vi "_builtins_arrange_diagram.vi"(8 "error in (no error)":errorcluster, 10 "Arrange":T1, 11 "VI Refnum in":refnum<vi>) -> (0 "error out":errorcluster, 3 "VI Refnum out":refnum<vi>)   [LabVIEW 2019, in "Script.lvlib"]
doc: "Arranges the selected diagram objects according to horizontal position and adjacent terminal location.\n\nCreated by: Ryan Pacini"
uses:
  Script.lvlib
  _builtins_arrange.ctl
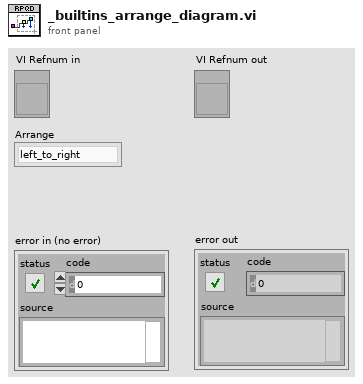
[diagram p1: front panel]
types:
  T1 = typedef "Script.lvlib/_builtins_arrange.ctl" = enum8{"left_to_right", "right_to_left"}
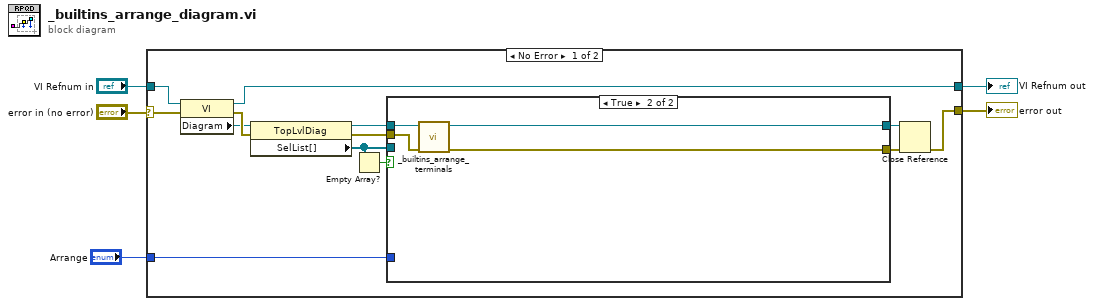
[diagram p0: block diagram]
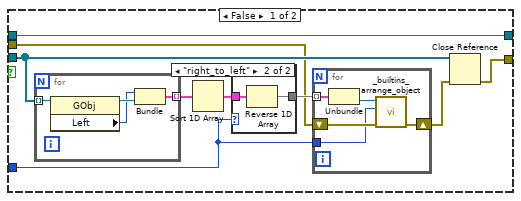
[diagram p2: hidden frame]
diagram:
  n1 = case shown="No Error" "error in (no error)" {
    selector: "error in (no error)" -> [w17 w44]
    tunnel: "VI Refnum in" -> [w18 w45]
    tunnel: [w10 w45] -> w4
    tunnel: [w6 w44] -> w2
    tunnel: "Arrange" -> [w14 _]
    frame No Error {
      n2 = property class="VI"(reference=w18, error in=w17) -> (reference out=w10:refnum<vi>, error out=w16:errorcluster, "Diagram"=w15:refnum<vi>)
      n3 = property class="TopLvlDiag"(reference=w15, error in=w16) -> (reference out=w9:refnum<vi>, error out=w11:errorcluster, "SelList[]"=w13:refnum<vi>[])
      n4 = Empty Array?(array=w13) -> (empty?=w12:bool)
      n5 = case shown="True" w12 {
        tunnel: [w24 w42] -> w7
        tunnel: w14 -> [w21 _]
        tunnel: w11 -> [w22 w43]
        tunnel: w13 -> [w23 _]
        tunnel: w9 -> [w19 w41]
        tunnel: [w19 w40] -> w8
        frame False {
          n6 = for {
            tunnel: w23 -> [w39] mode=indexing
            tunnel: [w36] -> w27 mode=indexing
            n7 = property class="GObj"(reference=w39) -> (reference out=w38:refnum<vi>, "Left"=w37:i32)  [unwired: 1 in, 1 out]
            n8 = Bundle("Left"=w37, w38) -> (w36:cluster{"Left":i32, refnum<vi>})  [unwired: 1 in]
          }
          n9 = Sort 1D Array(array=w27) -> (sorted array=w26:cluster{"Left":i32, refnum<vi>}[])
          n10 = case shown="\"right_to_left\"" w21 {
            tunnel: w26 -> [w28 w30]
            tunnel: [w28 w29] -> w25
            frame "left_to_right" {
            }
            frame "right_to_left" {
              n11 = Reverse 1D Array(array=w30) -> (reversed array=w29:cluster{"Left":i32, refnum<vi>}[])
            }
          }
          n12 = for {
            tunnel: w25 -> [w35] mode=indexing
            shift-right: [w33] -> w20
            shift-left: w22 -> [w32]
            tunnel: w21 -> [w31]
            n13 = Unbundle(w35) -> (w34:refnum<vi>)  [unwired: 1 out]
            n14 = call "_builtins_arrange_object.vi"("error in (no error)"=w32, "Arrange"=w31, "GObject in"=w34) -> ("error out"=w33:errorcluster)  [unwired: 6 in, 2 out]
          }
          n15 = Close Reference(reference=w23, error in (no error)=w20) -> (error out=w24:errorcluster)
        }
        frame True {
          n16 = call "_builtins_arrange_terminals.vi"("error in (no error)"=w43, "Diagram in"=w41) -> ("error out"=w42:errorcluster, "Diagram out"=w40:refnum<vi>)  [unwired: 8 in]
        }
      }
      n17 = Close Reference(reference=w8, error in (no error)=w7) -> (error out=w6:errorcluster)
    }
    frame Error {
    }
  }
  "VI Refnum out" <- w4
  "error out" <- w2
